vi "Leer_FicheroConfigBandejas_XML.vi"(8 "error in (no error)":errorcluster, 11 "XML File Path":path=path "C:/Trabajo_Robot/TFG_ROBOT/CONTROL_ROBOT/LABVIEW_ROBOT_MASTER") -> (0 "error out":errorcluster, 3 "Datos bandeja":T1={"Nº de columnas "=0, "Nº de filas "=0, "largo"=0, "ancho"=0, "nombre"="nombre", "Paso X (en mm)"=0.0, "Paso Y (en mm)"=0.0, "DISTANCIA SUELO A CHIP  "=0.0, "Nº de celdas totales"=0, "Distancia chips bandejas contiguas"=0.0})   [LabVIEW 2019, in "SHARED VI'S.lvlib"]
uses:
  LVPROJ_CREAR BANDEJAS/Type_defs/Data_Bandeja.ctl
  <vilib>/Utility/xml.llb/Read From XML File(string).vi
  SHARED VI'S.lvlib
panel:
  out "XML Elements":string
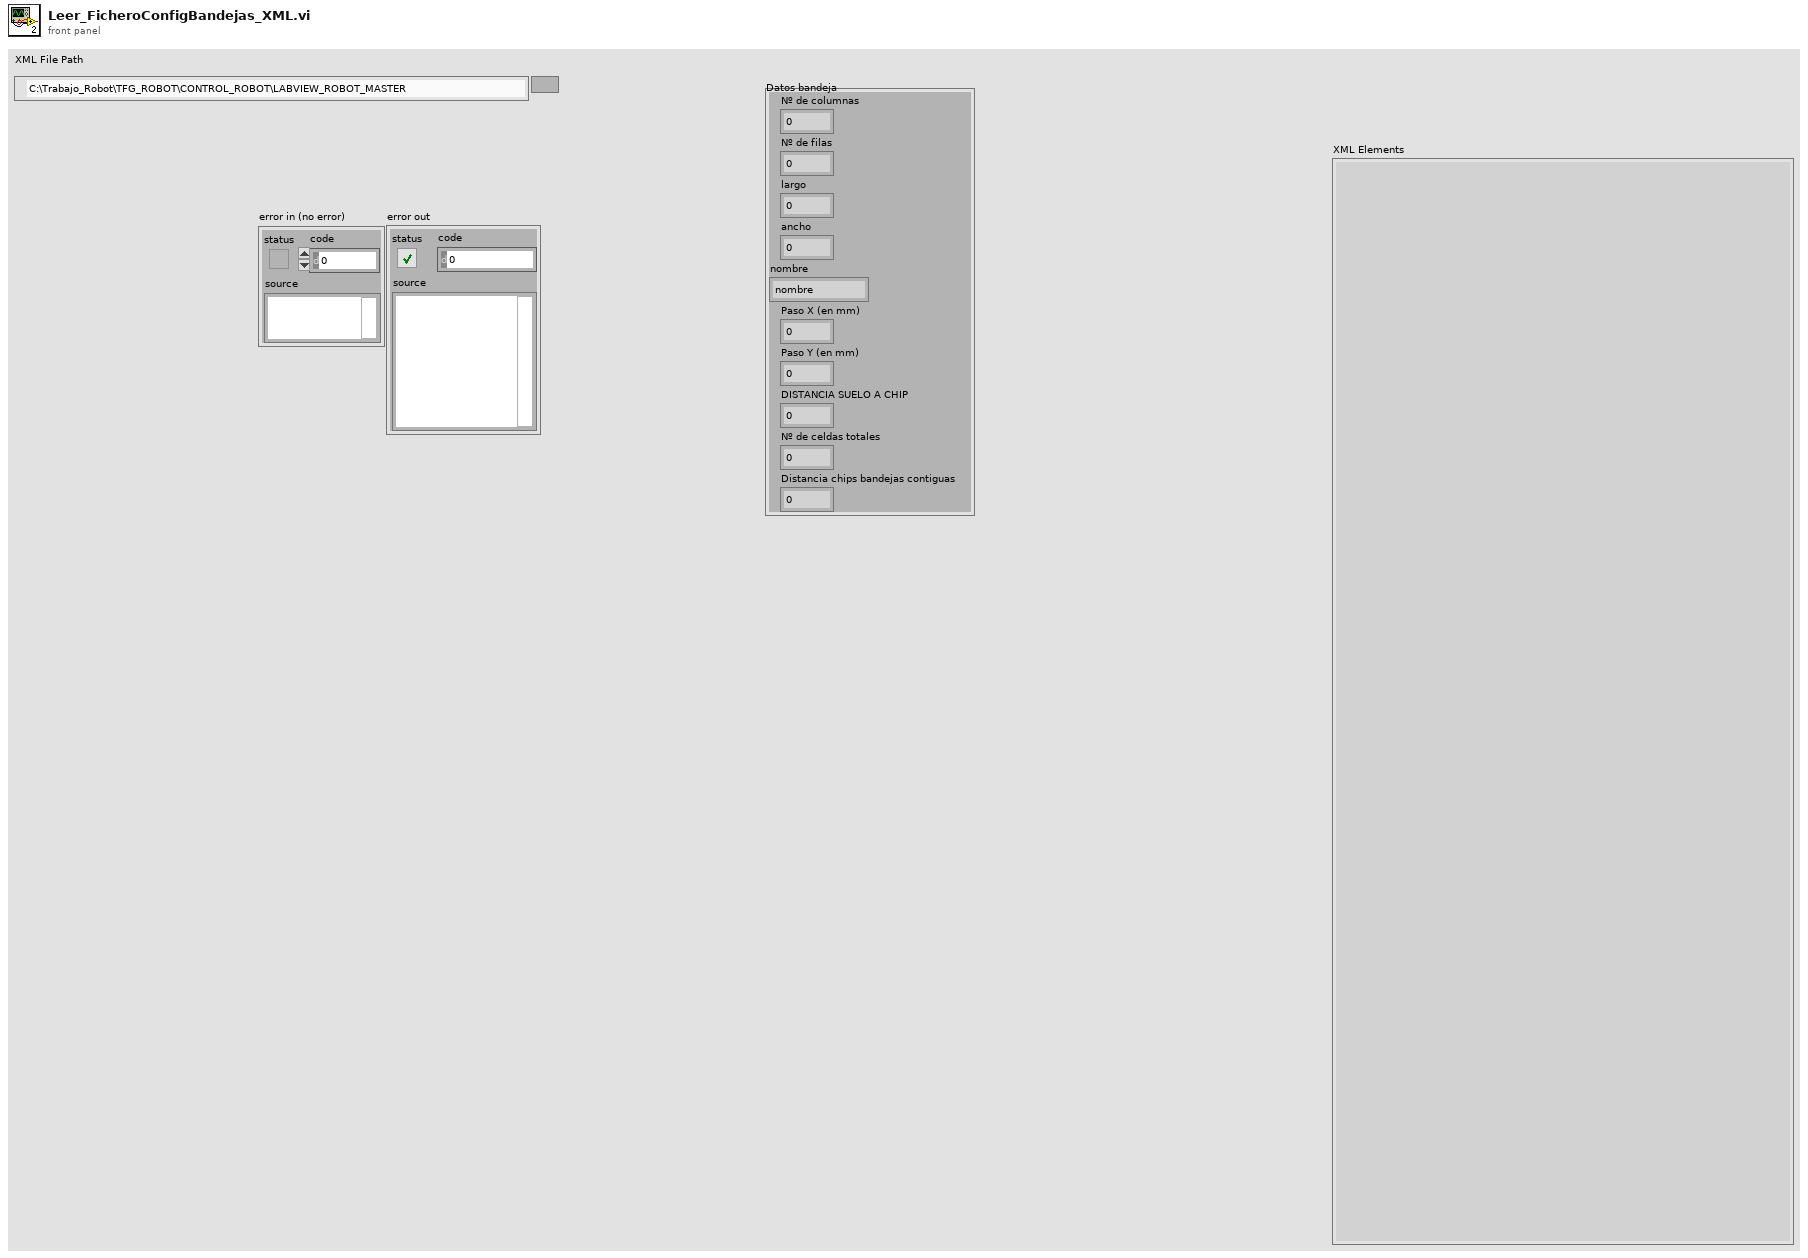
[diagram p1: front panel]
types:
  T1 = typedef "Data_Bandeja.ctl" = cluster{"Nº de columnas ":u32, "Nº de filas ":u32, "largo":u32, "ancho":u32, "nombre":string, "Paso X (en mm)":dbl, "Paso Y (en mm)":dbl, "DISTANCIA SUELO A CHIP  ":dbl, "Nº de celdas totales":u16, "Distancia chips bandejas contiguas":dbl}
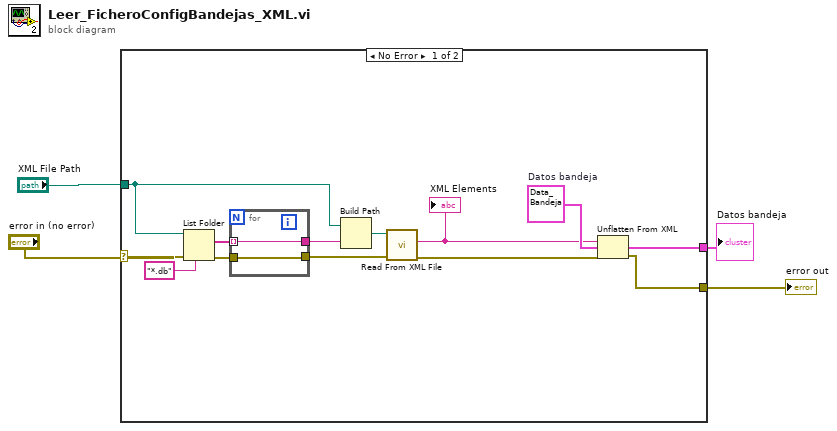
[diagram p0: block diagram]
diagram:
  n1 = case shown="No Error" "error in (no error)" {
    selector: "error in (no error)" -> [w10 _]
    tunnel: [w14 _] -> w3
    tunnel: [w13 _] -> w1
    tunnel: "XML File Path" -> [w7 _]
    frame No Error {
      w17 = T1 {"Nº de columnas "=0, "Nº de filas "=0, "largo"=0, "ancho"=0, "nombre"="nombre", "Paso X (en mm)"=0.0, "Paso Y (en mm)"=0.0, "DISTANCIA SUELO A CHIP  "=0.0, "Nº de celdas totales"=0, "Distancia chips bandejas contiguas"=0.0}  # Datos bandeja
      n2 = List Folder(path=w7, pattern="*.db", error in=w10) -> (filenames=w9:string[], error out=w6:errorcluster)  [unwired: 1 in, 2 out]
      n3 = for {
        tunnel: w9 -> [w19] mode=indexing
        tunnel: [w19] -> w8
        tunnel: [w18] -> w5
        tunnel: w6 -> [w18]
      }
      n4 = Build Path(base path=w7, name or relative path=w8) -> (appended path=w12:path)
      n5 = call-poly <vilib>:"Read From XML File.vi"("error in (no error)"=w5, "XML File Path"=w12) -> ("error out"=w15:errorcluster, "XML Elements"=w16:string)  [unwired: 7 in, 1 out]
      "XML Elements" <- w16
      n6 = Unflatten From XML(xml string=w16, type=w17, error in (no error)=w15) -> (value=w13:T1, error out=w14:errorcluster)
    }
    frame Error {
    }
  }
  "error out" <- w3
  "Datos bandeja" <- w1
